vi "Micro9.vi"(8 "errin":errorcluster caption="errout") -> (0 "errout":errorcluster={"status"=TRUE, "code"=0, "source"="PCAN_CHANNEL ILLEGAL"}, 1 "KO?":bool=TRUE, 2 "VISA OUT":T1={"Hitech"="COM97", "multi"="", "5520"="COM32", "3562"="COM24", "TakTak"="COM88"})   [LabVIEW 2020]
doc: "Ce vi il détecte la presence des équipements"
uses:
  Param_Sys.vi
panel:
  out "sortie d'erreur":errorcluster caption="errout"
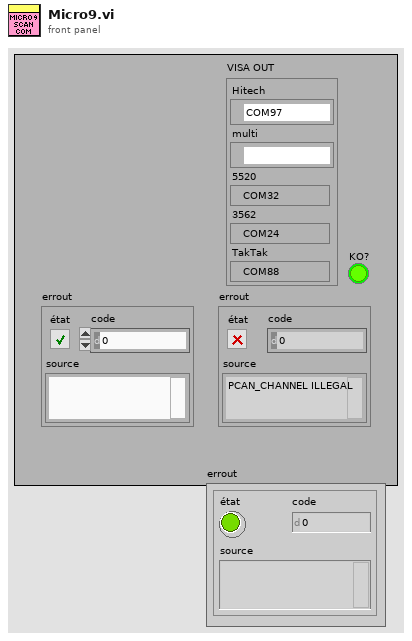
[diagram p1: front panel]
types:
  T1 = cluster{"Hitech":refnum<visa-resource-name>, "multi":refnum<visa-resource-name>, "5520":refnum<visa-resource-name>, "3562":refnum<visa-resource-name>, "TakTak":refnum<visa-resource-name>}
  T2 = cluster{"Hitech":string, "multi":string, "5520":string, "3562":string, "TakTak":string}
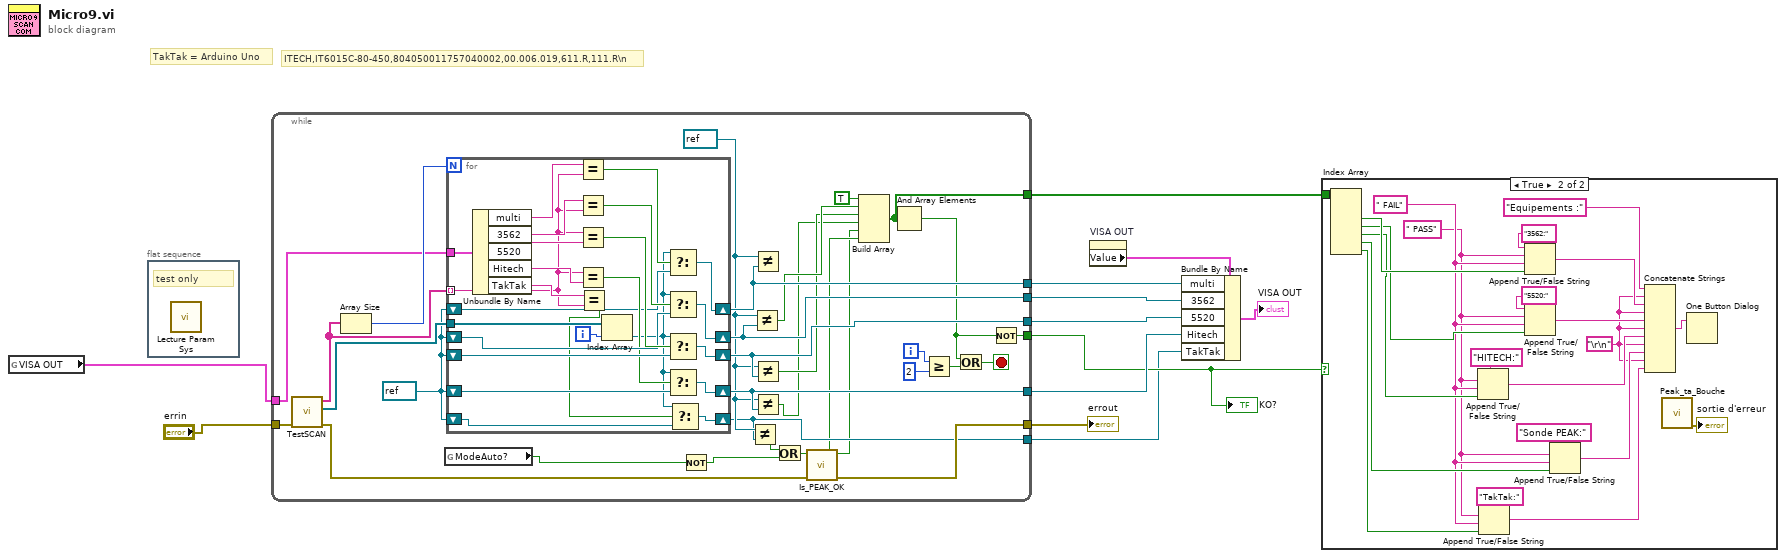
[diagram p0: block diagram]
diagram:
  # "TakTak = Arduino Uno"
  # "ITECH,IT6015C-80-450,804050011757040002,00.006.019,611.R,111.R\\n"
  n1 = global read "Param_Sys.vi" "VISA OUT"() -> (w1:T2)
  n2 = flat-sequence {
    frame #0 {
      # "test only"
      n3 = call "Lecture Param Sys.vi"() -> ()  [unwired: 11 in, 1 out]
    }
  }
  n4 = while {
    tunnel: [w28] -> w11
    tunnel: [w27] -> w10
    tunnel: "errin" -> [w41]
    tunnel: [w26] -> w9
    tunnel: [w36] -> w5
    tunnel: [w29] -> w12
    tunnel: w1 -> [w33]
    tunnel: [w32] -> w6
    tunnel: [w24] -> w4
    tunnel: [w19] -> w3
    i -> [w35]
    stop <- w38 stop-if-true
    w25 = refnum<visa-resource-name> refnum ("x")
    w30 = refnum<visa-resource-name> refnum ("VISA resource name out")
    n5 = call "TestSCAN.vi"("errin"=w41) -> ("error out"=w31:errorcluster, "Tableau 2"=w39:refnum<visa-resource-name>[], "Tableau"=w40:string[])  [unwired: 8 in]
    n6 = Array Size(array=w40) -> (size(s)=w42:i32)
    n7 = global read "Param_Sys.vi" "ModeAuto?"() -> (w14:bool)
    n8 = for {
      N: w42 -> [_]
      shift-right: [w63] -> w28
      shift-left: w30 -> [w61]
      shift-right: [w62] -> w27
      shift-left: w30 -> [w60]
      tunnel: w40 -> [w47] mode=indexing
      tunnel: w39 -> [w66]
      shift-right: [w58] -> w26
      shift-left: w30 -> [w57]
      shift-right: [w54] -> w29
      shift-left: w30 -> [w55]
      tunnel: w33 -> [w53]
      shift-right: [w43] -> w24
      shift-left: w30 -> [w44]
      i -> [w65]
      n9 = Unbundle By Name(w53) -> ("multi"=w52:string, "3562"=w51:string, "5520"=w50:string, "Hitech"=w49:string, "TakTak"=w48:string)
      n10 = Equal?(x=w52, y=w47) -> (x = y?=w56:bool)
      n11 = Equal?(x=w51, y=w47) -> (x = y?=w64:bool)
      n12 = Equal?(x=w47, y=w50) -> (x = y?=w67:bool)
      n13 = Equal?(x=w47, y=w49) -> (x = y?=w59:bool)
      n14 = Equal?(x=w48, y=w47) -> (x = y?=w46:bool)
      n15 = Index Array(array=w66, index=w65) -> (element=w45:refnum<visa-resource-name>)
      n16 = Select(t=w45, s=w56, f=w55) -> (s? t:f=w54:refnum<visa-resource-name>)
      n17 = Select(t=w45, s=w64, f=w61) -> (s? t:f=w63:refnum<visa-resource-name>)
      n18 = Select(t=w45, s=w67, f=w60) -> (s? t:f=w62:refnum<visa-resource-name>)
      n19 = Select(t=w45, s=w59, f=w57) -> (s? t:f=w58:refnum<visa-resource-name>)
      n20 = Select(t=w45, s=w46, f=w44) -> (s? t:f=w43:refnum<visa-resource-name>)
    }
    n21 = Not(x=w14) -> (.not. x?=w15:bool)
    n22 = Not Equal?(x=w25, y=w24) -> (x != y?=w17:bool)
    n23 = Not Equal?(x=w25, y=w28) -> (x != y?=w23:bool)
    n24 = Not Equal?(x=w25, y=w29) -> ()  [unwired: 1 out]
    n25 = Not Equal?(x=w25, y=w27) -> (x != y?=w22:bool)
    n26 = Not Equal?(x=w25, y=w26) -> (x != y?=w21:bool)
    n27 = Or(x=w17, y=w15) -> (x .or. y?=w16:bool)
    n28 = call <userlib>:"Is_PEAK_OK.vi"("errin"=w31) -> ("error out"=w32:errorcluster, "x = 0 ?"=w13:bool)  [unwired: 9 in]
    n29 = Build Array(TRUE ("élément"), w23, w22, w21, w13, w16) -> (w19:bool[])
    n30 = And Array Elements(Boolean array=w19) -> (logical AND=w20:bool)
    n31 = Greater Or Equal?(x=w35, y=2) -> (x >= y?=w37:bool)
    n32 = Or(x=w20, y=w37) -> (x .or. y?=w38:bool)
    n33 = Not(x=w20) -> (.not. x?=w36:bool)
  }
  "KO?" <- w5
  "errout" <- w6
  n34 = property on="VISA OUT" class="Clust (strict)"() -> ("Value"=w8:T1)  [unwired: 2 in, 2 out]
  n35 = Bundle By Name(cluster=w8, "multi"=w12, "3562"=w11, "5520"=w10, "Hitech"=w9, "TakTak"=w4) -> (→"VISA OUT":T1)
  n36 = case shown="True" w5 {
    tunnel: w3 -> [_ w76]
    frame False {
    }
    frame True {
      w78 = "\r\n"
      w69 = " PASS" ("chaîne faux")
      w70 = " FAIL" ("chaîne faux")
      n37 = Index Array(array=w76) -> (element #2=w75:bool, element #3=w74:bool, element #4=w73:bool, element #5=w72:bool, element #6=w71:bool)  [unwired: 6 in, 1 out]
      n38 = Append True/False String(1:w73, 2:w70, 3:w69, 4:"HITECH:" ("chaîne (\"\")")) -> (0:w82:string)
      n39 = Append True/False String ("Ajouter la chaîne Vrai/Faux")(1:w71, 2:w70, 3:w69, 4:"TakTak:" ("chaîne (\"\")")) -> (0:w77:string)
      n40 = Append True/False String(1:w75, 2:w70, 3:w69, 4:"3562:" ("chaîne (\"\")")) -> (0:w84:string)
      n41 = Append True/False String(1:w74, 2:w70, 3:w69, 4:"5520:" ("chaîne (\"\")")) -> (0:w83:string)
      n42 = Append True/False String(1:w72, 2:w70, 3:w69, 4:"Sonde PEAK:" ("chaîne (\"\")")) -> (0:w81:string)
      n43 = Concatenate Strings("Equipements :" ("chaîne"), w78, w84, w78, w83, w78, w82, w78, w81, w78, w77) -> (w80:string)
      n44 = call <userlib>:"Peak_ta_Bouche.vi"() -> ("sortie d'erreur"=→"sortie d'erreur":errorcluster)  [unwired: 11 in]
      n45 = One Button Dialog(message=w80) -> ()  [unwired: 1 in, 1 out]
    }
  }
